vi "Start Engine.vi"(7 "Engine Type":refnum<class "LQCoreEngine.lvclass">, 8 "Error In":errorcluster) -> (0 "Error Out":errorcluster, 3 "New Engine":refnum<class "LQCoreEngine.lvclass">)   [LabVIEW 2013, in "Template.lvlib" / "LQCoreEngine.lvclass"]
uses:
  LQCoreEngine.lvclass
  Internal/LQIdentity Registry Action.ctl
  LQIdentity/LQIdentity.lvclass/LQIdentity.ctl
  _Private/Global Quit Event Holder.vi
  Template.lvlib
  LQIdentity/LQIdentity.lvclass
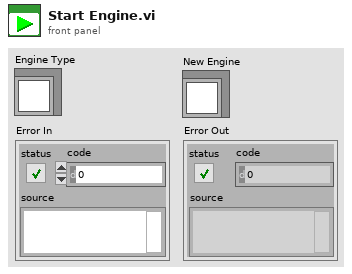
[diagram p1: front panel]
types:
  T1 = typedef "Template.lvlib/LQCoreEngine.lvclass/LQIdentity Registry Action.ctl" = enum16{"Init", "Register LQIdentity", "Get LQIdentity Info", "Deregister LQIdentity"}
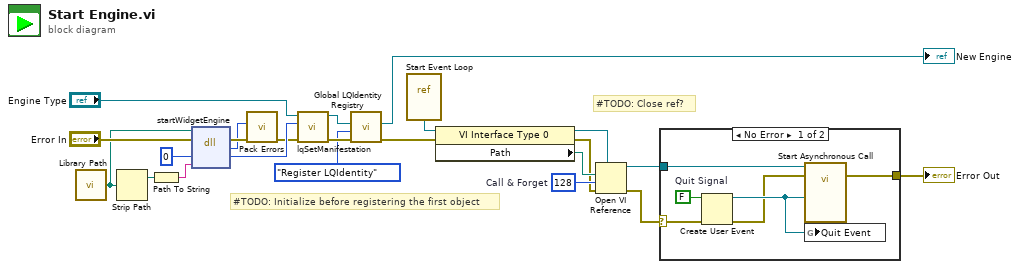
[diagram p0: block diagram]
diagram:
  w22 = 128  # Call & Forget
  # "#TODO: Initialize before registering the first object"
  # "#TODO: Close ref?"
  n1 = call "Library Path.vi"() -> ("Library Path"=w17:path)
  n2 = Strip Path(path=w17) -> (stripped path=w16:path)  [unwired: 1 out]
  n3 = Path To String(path=w16) -> (string=w15:string)
  n4 = dll-call lib="?" fn="startWidgetEngine"(path in=w17, error in="Error In", "_retVal"=u64 0, "pluginDir"=w15) -> (error out=w14:errorcluster, "errorCode"=w13:i32, "_retVal"=w7:u64)  [unwired: 2 in, 1 out]
  n5 = call "Pack Errors.vi"("Error In"=w14, "Error Code"=w13) -> ("Error Out"=w6:errorcluster)  [unwired: 9 in]
  n6 = call "lqSetManifestation.vi"("Error In"=w6, "Manifestation"=w7, "LQIdentity in"="Engine Type") -> ("Error Out"=w9:errorcluster, "LQIdentity out"=w10:refnum<class "LQCoreEngine.lvclass">)  [unwired: 7 in]
  n7 = call "Global LQIdentity Registry.vi"("Error In"=w9, "Registry Action"=LQIdentity_Registry_Action."Register LQIdentity", "LQIdentity Info In"=w10) -> ("Error Out"=w1:errorcluster, "LQIdentity Info Out"=→"New Engine":refnum<class "LQCoreEngine.lvclass">)  [unwired: 7 in]
  n8 = vi-ref "Start Event Loop.vi"() -> (w19:refnum<vi>)
  n9 = property class="VI Interface Type 0"(reference=w19, error in=w1) -> (reference out=w20:refnum<vi>, error out=w18:errorcluster, "Path"=w21:path)
  n10 = Open VI Reference(type specifier VI Refnum (for type only)=w20, vi path=w21, options=w22, error in (no error)=w18) -> (vi reference=w4:refnum<vi>, error out=w12:errorcluster)  [unwired: 2 in]
  n11 = case shown="No Error" w12 {
    selector: w12 -> [w28 w30]
    tunnel: w4 -> [w27 _]
    tunnel: [w24 w30] -> w3
    frame No Error {
      w29 = FALSE  # Quit Signal
      n12 = Create User Event(user event datatype=w29, error in=w28) -> (user event=w26:refnum<user-event>, error out=w25:errorcluster)
      n13 = call-by-ref "Start Asynchronous Call"(reference=w27, error in=w25, "Quit Event"=w26) -> (error out=w24:errorcluster)  [unwired: 11 in, 1 out]
      n14 = global write "Global Quit Event Holder.vi" "Quit Event"(w26) -> ()
    }
    frame Error {
    }
  }
  "Error Out" <- w3
